vi "Update_File_Name.vi"(3 "Number of Channels":i32, 4 "New File":bool, 5 "File Path IN":path) -> (0 "Text Image Data Path":path, 1 "File References":path[](array[path]), 2 "File Path OUT":path)   [LabVIEW 2016]
panel:
  # "Copyright (C) 2020 Edward S Allgeyer\n\nRedistribution and use in source and binary forms, with or without\nmodification, are permitted provided that the following conditions\nare met:\n\n1. Redistributions of source code must retain the above copyright\n   notice, this list of conditions and the following disclaimer.\n\n2. Redistributions in binary form must reproduce the above copyright\n   notice, this list of conditions and the following disclaimer in\n   the documentation and/or other materials provided with the\n   distribution.\n\n3. Neither the name of the copyright holder nor the names of its\n   contributors may be used to endorse or promote products derived\n   from this software without specific prior written permission.\n\nTHIS SOFTWARE IS PROVIDED BY THE COPYRIGHT HOLDERS AND CONTRIBUTORS\n\"AS IS\" AND ANY EXPRESS OR IMPLIED WARRANTIES, INCLUDING, BUT NOT\nLIMITED TO, THE IMPLIED WARRANTIES OF MERCHANTABILITY AND FITNESS\nFOR A PARTICULAR PURPOSE ARE DISCLAIMED. IN NO EVENT SHALL THE\nCOPYRIGHT HOLDER OR CONTRIBUTORS BE LIABLE FOR ANY DIRECT, INDIRECT,\nINCIDENTAL, SPECIAL, EXEMPLARY, OR CONSEQUENTIAL DAMAGES (INCLUDING,\nBUT NOT LIMITED TO, PROCUREMENT OF SUBSTITUTE GOODS OR SERVICES;\nLOSS OF USE, DATA, OR PROFITS; OR BUSINESS INTERRUPTION) HOWEVER\nCAUSED AND ON ANY THEORY OF LIABILITY, WHETHER IN CONTRACT, STRICT\nLIABILITY, OR TORT (INCLUDING NEGLIGENCE OR OTHERWISE) ARISING IN\nANY WAY OUT OF THE USE OF THIS SOFTWARE, EVEN IF ADVISED OF THE\nPOSSIBILITY OF SUCH DAMAGE."
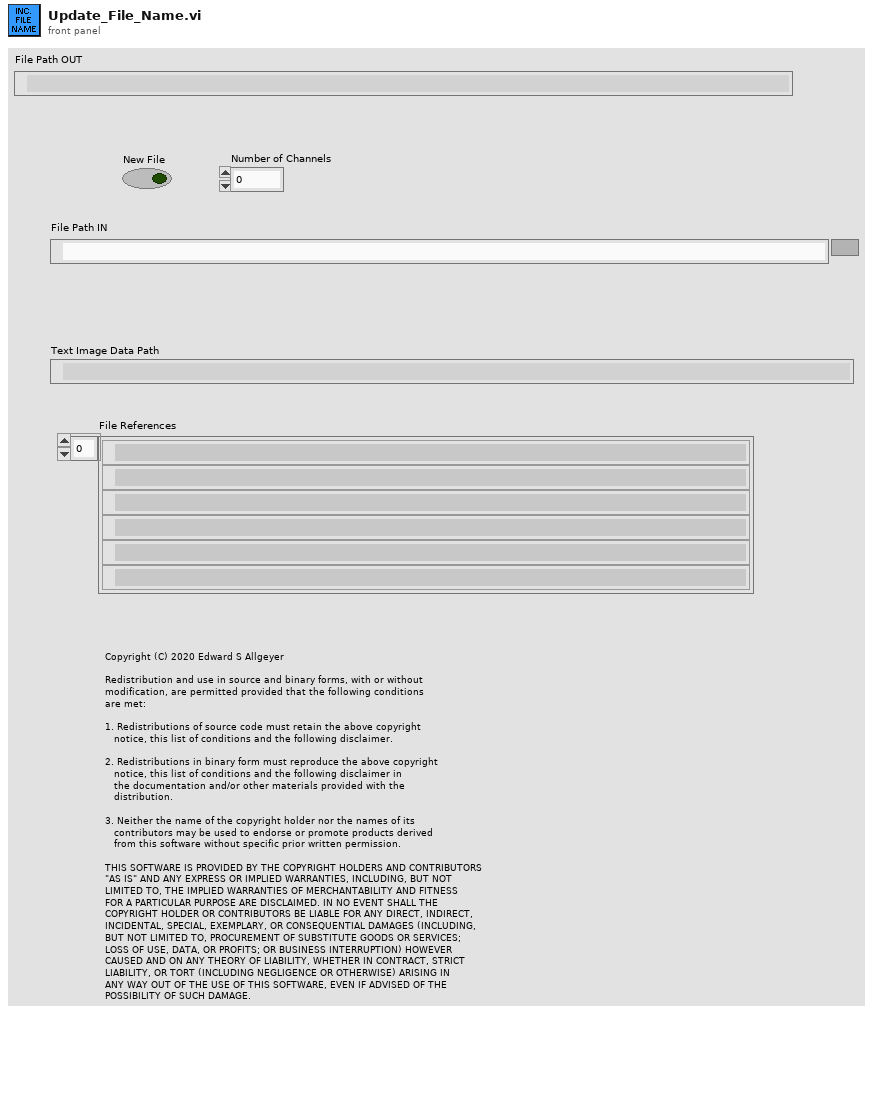
[diagram p1: front panel]
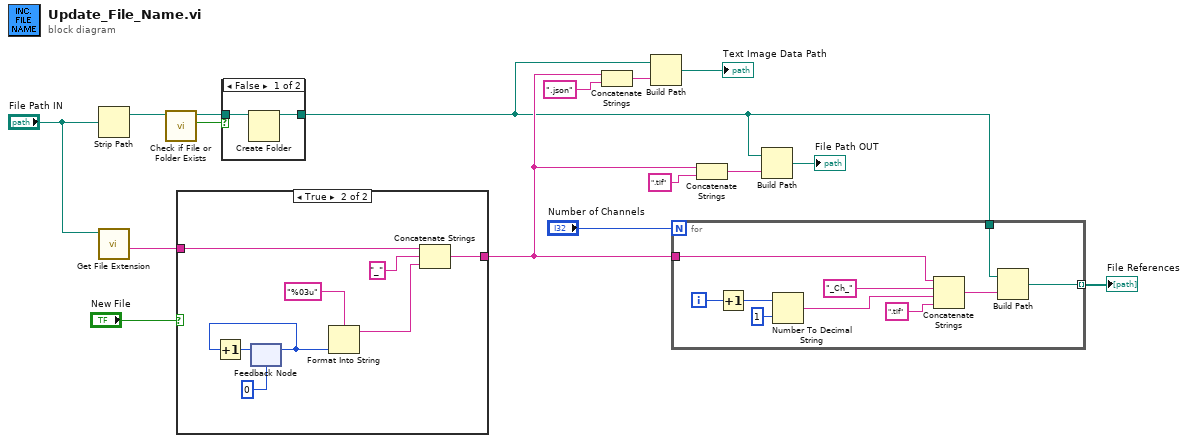
[diagram p0: block diagram]
diagram:
  n1 = Strip Path(path="File Path IN") -> (stripped path=w4:path)  [unwired: 1 out]
  n2 = call <vilib>:"Get File Extension.vi"("file"="File Path IN") -> ("filename without extension"=w16:string)  [unwired: 6 in, 4 out]
  n3 = call <vilib>:"Check if File or Folder Exists.vi"("path"=w4) -> ("file or folder exists?"=w3:bool, "dup path"=w2:path)  [unwired: 8 in, 1 out]
  n4 = case shown="True" "New File" {
    tunnel: w16 -> [w17 w23]
    tunnel: [w17 w18] -> w7
    frame False {
    }
    frame True {
      n5 = feedback #1(u16 0) -> (w21:u16)
      n6 = Increment(x=w21) -> (x+1=w24:u16)
      n7 = feedback-in #1(w24) -> ()
      n8 = Format Into String(format string="%03u", w21) -> (resulting string=w19:string)  [unwired: 2 in, 1 out]
      n9 = Concatenate Strings(w23, "_", w19) -> (w18:string)
    }
  }
  n10 = case shown="False" w3 {
    tunnel: w2 -> [w27 w28]
    tunnel: [w26 w28] -> w1
    frame False {
      n11 = Create Folder(path (use dialog)=w27) -> (created path=w26:path)  [unwired: 2 in, 2 out]
    }
    frame True {
    }
  }
  n12 = Concatenate Strings(w7, ".json" ("string")) -> (w13:string)
  n13 = Build Path(base path=w1, name or relative path=w13) -> (appended path=→"Text Image Data Path":path)
  n14 = for {
    N: "Number of Channels" -> [_]
    tunnel: w7 -> [w35]
    tunnel: w1 -> [w31]
    tunnel: [w29] -> w9 mode=indexing
    i -> [w38]
    n15 = Increment(x=w38) -> (x+1=w33:i32)
    n16 = Number To Decimal String(number=w33, width (-)=i16 1) -> (decimal integer string=w32:string)
    n17 = Concatenate Strings(w35, "_Ch_" ("string"), w32, ".tif" ("string")) -> (w30:string)
    n18 = Build Path(base path=w31, name or relative path=w30) -> (appended path=w29:path)
  }
  "File References" <- w9
  n19 = Concatenate Strings(w7, ".tif" ("string")) -> (w6:string)
  n20 = Build Path(base path=w1, name or relative path=w6) -> (appended path=→"File Path OUT":path)
